vi "NIST Time Synch.vi"(4 "error in (no error)":errorcluster) -> (0 "error out":errorcluster, 1 "Erro>24H":bool, 3 "UTC Date Time":timestamp)   [LabVIEW 2018]
uses:
  <vilib>/Utility/miscctls.llb/LVDateTimeRec.ctl
panel:
  out "x-y":dbl
  out "PC Date Time":timestamp
  out "output cluster":T1
  out "empty?":bool
  out "data out":string
  out "16bit integer":cluster{i16, i16, i16, i16, i16, i16}
  out "Time Server IP Address (129.6.15.29)":string="129.6.15.29"
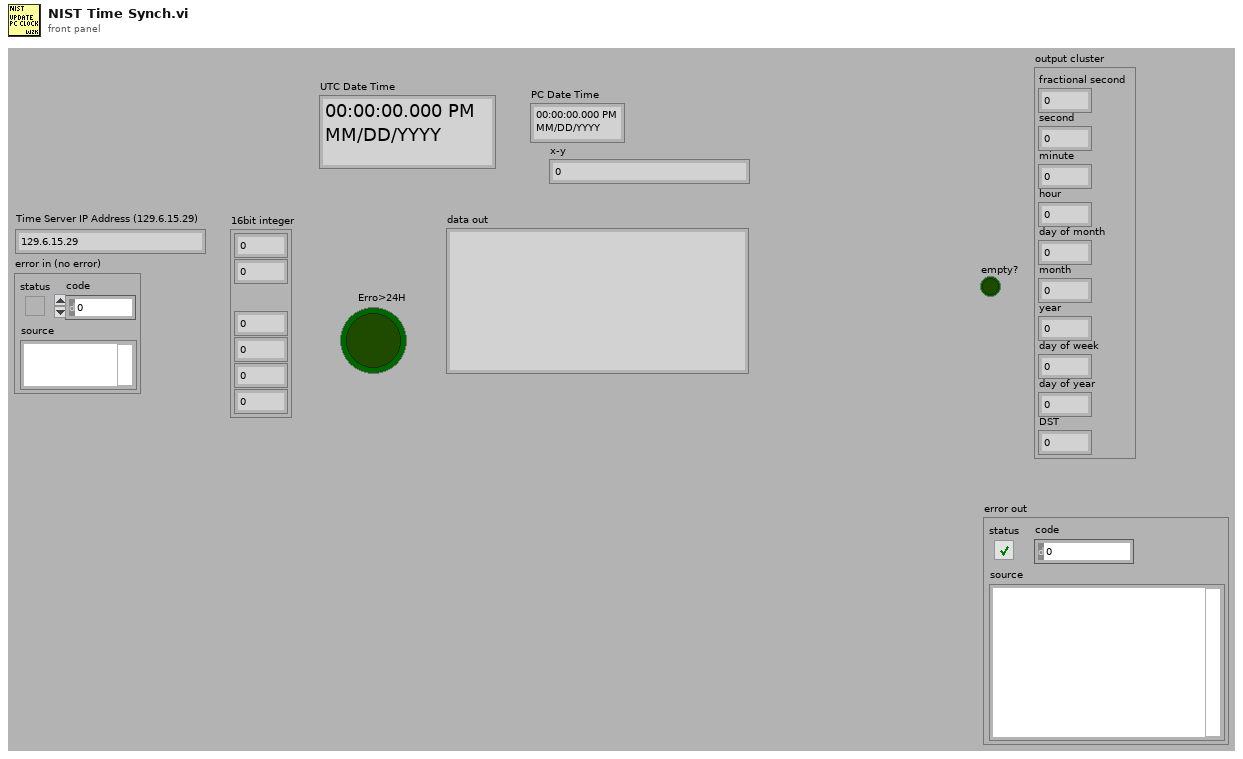
[diagram p1: front panel]
types:
  T1 = typedef "LVDateTimeRec.ctl" = cluster{"fractional second":dbl, "second":i32, "minute":i32, "hour":i32, "day of month":i32, "month":i32, "year":i32, "day of week":i32, "day of year":i32, "DST":i32}
  T2 = enum16{"Standard", "Buffered", "CRLF", "Immediate"}
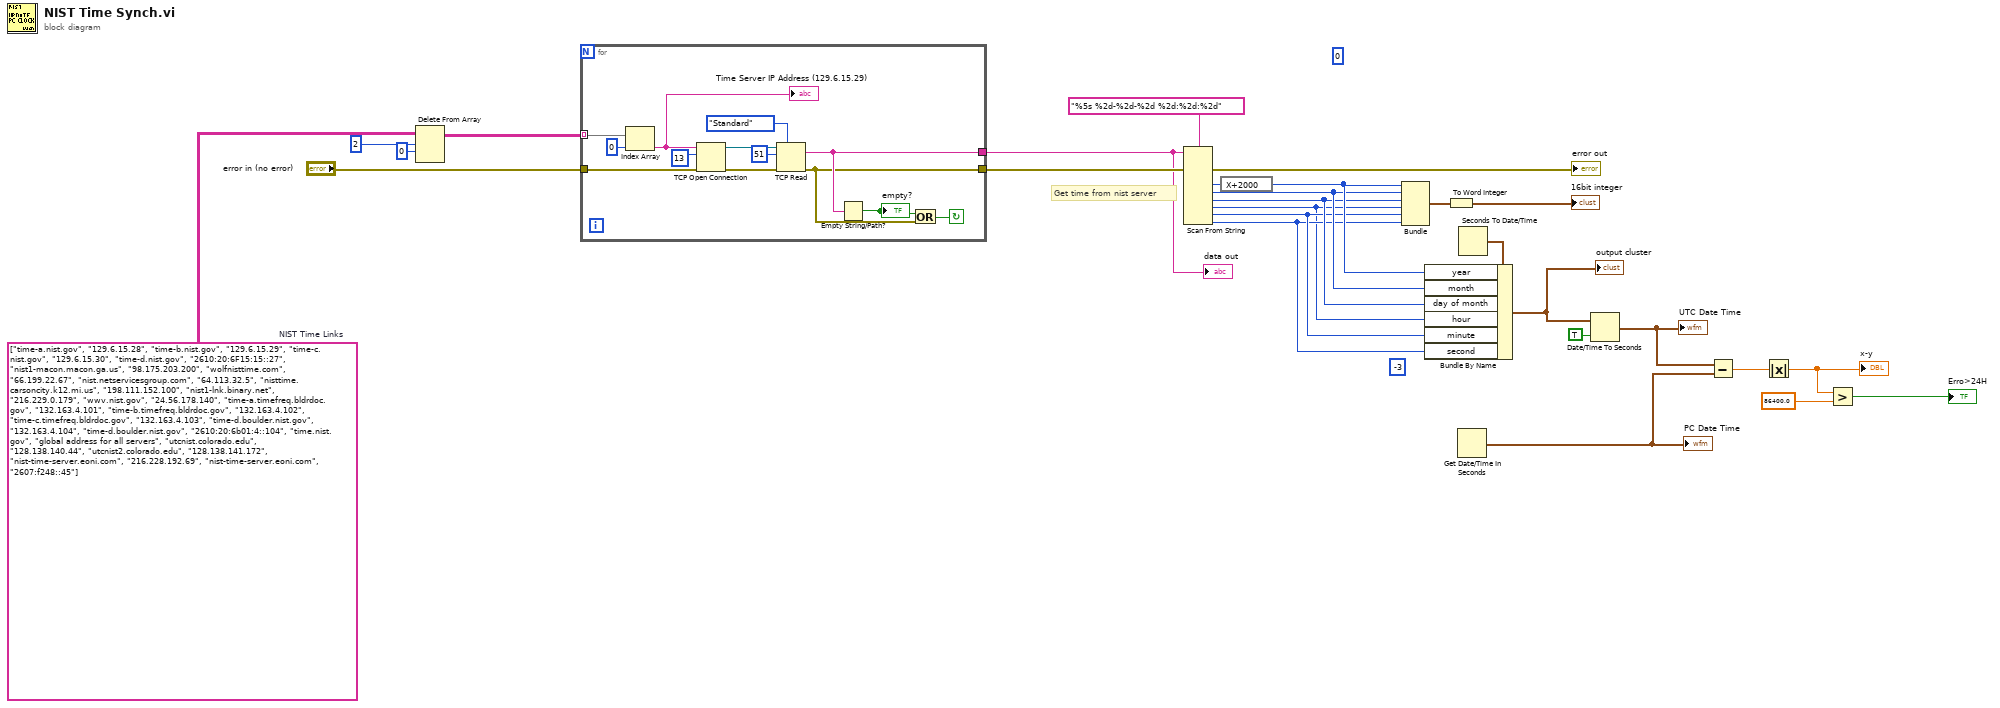
[diagram p0: block diagram]
diagram:
  (unwired) -3 ("DST")
  w12 = string[][] [["time-a.nist.gov", "129.6.15.28"], ["time-b.nist.gov", "129.6.15.29"], ["time-c.nist.gov", "129.6.15.30"], ["time-d.nist.gov", "2610:20:6F15:15::27"], ["nist1-macon.macon.ga.us", "98.175.203.200"], ["wolfnisttime.com", "66.199.22.67"], ["nist.netservicesgroup.com", "64.113.32.5"], ["nisttime.carsoncity.k12.mi.us", "198.111.152.100"], ["nist1-lnk.binary.net", "216.229.0.179"], ["wwv.nist.gov", "24.56.178.140"], ["time-a.timefreq.bldrdoc.gov", "132.163.4.101"], ["time-b.timefreq.bldrdoc.gov", "132.163.4.102"], ["time-c.timefreq.bldrdoc.gov", "132.163.4.103"], ["time-d.boulder.nist.gov", "132.163.4.104"], ["time-d.boulder.nist.gov", "2610:20:6b01:4::104"], ["time.nist.gov", "global address for all servers"], ["utcnist.colorado.edu", "128.138.140.44"], ["utcnist2.colorado.edu", "128.138.141.172"], ["nist-time-server.eoni.com", "216.228.192.69"], ["nist-time-server.eoni.com", "2607:f248::45"]]  # NIST Time Links
  (unwired) 0
  # "Get time from nist server"
  n1 = Delete From Array(array=w12, length=2, index (row)=0) -> (array with subset deleted=w9:string[][])  [unwired: 1 in, 1 out]
  n2 = for {
    tunnel: w9 -> [w39] mode=indexing
    tunnel: [w30] -> w16
    tunnel: [w33] -> w15
    tunnel: "error in (no error)" -> [w29]
    stop <- w31 continue-if-true
    n3 = Index Array(array=w39, index=0) -> (element=w28:string)
    "Time Server IP Address (129.6.15.29)" <- w28
    n4 = TCP Open Connection(address=w28, remote port or service name=u16 13 ("port"), error in (no error)=w29) -> (connection ID=w35:refnum<k5>, error out=w34:errorcluster)  [unwired: 2 in]
    n5 = TCP Read(connection ID=w35, bytes to read=51, error in (no error)=w34, 7:T2."Standard" ("mode (standard)")) -> (data out=w33:string, error out=w30:errorcluster)  [unwired: 1 in, 1 out]
    n6 = Empty String/Path?(string/path=w33) -> (empty?=w32:bool)
    "empty?" <- w32
    n7 = Or(x=w32, y=w30) -> (x .or. y?=w31:bool)
  }
  "data out" <- w15
  n8 = Scan From String(format string="%5s %2d-%2d-%2d %2d:%2d:%2d", input string=w15, error in=w16) -> (error out=→"error out":errorcluster, output 2=w26:i32, output 3=w22:i32, output 4=w21:i32, output 5=w17:i32, output 6=w19:i32, output 7=w18:i32)  [unwired: 9 in, 2 out]
  n9 = expression code="X+2000"(w26) -> (w23:i32)
  n10 = Bundle(w23, w22, w21, w17, w19, w18) -> (w25:cluster{i32, i32, i32, i32, i32, i32})  [unwired: 1 in]
  n11 = To Word Integer(number=w25) -> (16bit integer=→"16bit integer":cluster{i16, i16, i16, i16, i16, i16})
  n12 = Get Date/Time In Seconds() -> (seconds since 1Jan1904=w6:timestamp)
  "PC Date Time" <- w6
  n13 = Seconds To Date/Time() -> (date time rec=w8:T1)  [unwired: 2 in]
  n14 = Bundle By Name(cluster=w8, "year"=w23, "month"=w22, "day of month"=w21, "hour"=w17, "minute"=w19, "second"=w18) -> (w20:T1)
  "output cluster" <- w20
  n15 = Date/Time To Seconds(1:TRUE ("is UTC (F)"), 2:w20) -> (0:w7:timestamp)
  "UTC Date Time" <- w7
  n16 = Subtract(x=w7, y=w6) -> (x-y=w5:dbl)
  n17 = Absolute Value(x=w5) -> (abs(x)=w4:dbl)
  "x-y" <- w4
  n18 = Greater?(x=w4, y=86400.0) -> (0:→"Erro>24H":bool)
